vi "1D Quadrature Integrand for Gated Decay.vi"(10 "data":variant, 11 "X":dbl[](array[numeric])) -> (0 "Error Out":errorcluster, 3 "F(X)":dbl[](array[numeric]))   [LabVIEW 2019]
doc: "This template is the starting point for creating a function that is the integrand evaluation to be passed to the Quadrature.vi."
uses:
  Gate & Decay Parameters.ctl
  Gate Type.ctl
  IRF Model.ctl
  XY Plot Data.ctl
  a549e530-db8e-4861-84b1-6abd4ac2432e.vi/28aad339-045a-48ec-96ec-2fcecac66ea0.vi
  <vilib>/Utility/error.llb/Error Cluster From Error Code.vi
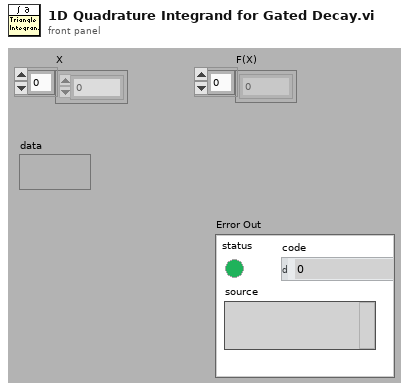
[diagram p1: front panel]
types:
  T1 = typedef "Gate & Decay Parameters.ctl" = cluster{"W":dbl, "T":dbl, "tau":dbl, "t_0":dbl, "Gate Type":T2, "t_i":dbl, "sR":dbl, "sF":dbl, "s":dbl, "Reversed Sawtooth":bool, "IRF Model":T3, "IRF Parameter 1":dbl, "User-defined Gate":T4, "Type of User-defined Function":enum32{"Gate", "IRF"}}
  T2 = typedef "Gate Type.ctl" = enum16{"Square", "Finite Edge Square", "Finite Edge, Tilted Top Square", "Triangle", "Sawtooth", "User-defined"}
  T3 = typedef "IRF Model.ctl" = enum16{"Dirac", "Exponential"}
  T4 = typedef "XY Plot Data.ctl" = cluster{"X Array":dbl[], "Y Array":dbl[]}
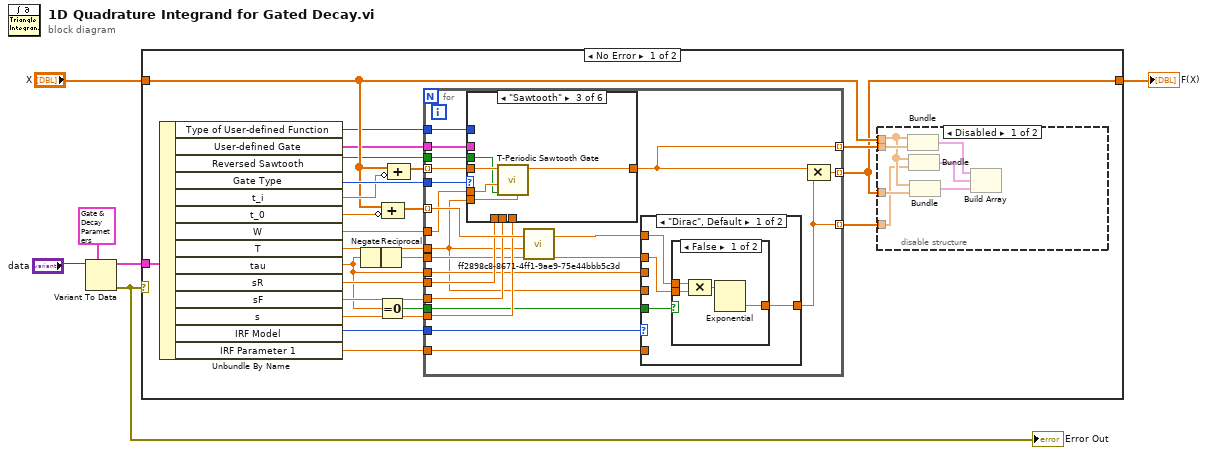
[diagram p0: block diagram]
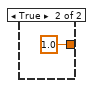
[diagram p3: hidden frame]
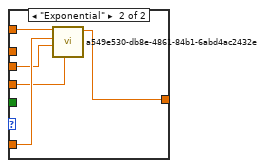
[diagram p4: hidden frame]
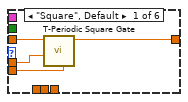
[diagram p5: hidden frame]
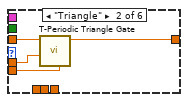
[diagram p6: hidden frame]
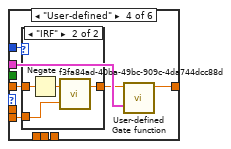
[diagram p7: hidden frame]
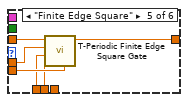
[diagram p9: hidden frame]
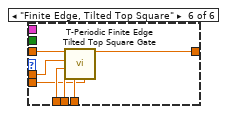
[diagram p10: hidden frame]
diagram:
  n1 = Variant To Data(type=T1 {"W"=0.0, "T"=0.0, "tau"=0.0, "t_0"=0.0, "Gate Type"=enum."Square", "t_i"=0.0, "sR"=0.0, "sF"=0.0, "s"=0.0, "Reversed Sawtooth"=FALSE, "IRF Model"=enum."Dirac", "IRF Parameter 1"=0.0, "User-defined Gate"={"X Array"=[], "Y Array"=[]}, "Type of User-defined Function"=enum."Gate"} ("Gate & Decay Parameters"), Variant="data") -> (data=w3:T1, error out=w2:errorcluster)  [unwired: 1 in]
  "Error Out" <- w2
  n2 = case shown="No Error" w2 {
    tunnel: "X" -> [w23 _]
    tunnel: w3 -> [w9 _]
    tunnel: [w7 _] -> w1
    frame No Error {
      n3 = Unbundle By Name(w9) -> ("Type of User-defined Function"=w8:enum32{"Gate", "IRF"}, "User-defined Gate"=w12:T4, "Reversed Sawtooth"=w15:bool, "Gate Type"=w29:T2, "t_i"=w28:dbl, "t_0"=w26:dbl, "W"=w21:dbl, "T"=w30:dbl, "tau"=w11:dbl, "sR"=w18:dbl, "sF"=w17:dbl, "s"=w16:dbl, "IRF Model"=w14:T3, "IRF Parameter 1"=w13:dbl)
      n4 = Negate(x=w11) -> (-x=w20:dbl)
      n5 = Reciprocal(x=w20) -> (1/x=w19:dbl)
      n6 = Equal To 0?(x=w11) -> (x = 0?=w10:bool)
      n7 = Compound Arithmetic op=ADD(w23, invert w26) -> (w25:dbl[])
      n8 = Compound Arithmetic op=ADD(w23, invert w28) -> (w27:dbl[])
      n9 = for {
        tunnel: w30 -> [w39]
        tunnel: w19 -> [w41]
        tunnel: w25 -> [w53] mode=indexing
        tunnel: w27 -> [w57] mode=indexing
        tunnel: w29 -> [w56]
        tunnel: [w55] -> w7 mode=indexing
        tunnel: [w54] -> w24 mode=indexing
        tunnel: [w51] -> w22 mode=indexing
        tunnel: w21 -> [w52]
        tunnel: w18 -> [w50]
        tunnel: w17 -> [w49]
        tunnel: w16 -> [w48]
        tunnel: w15 -> [w47]
        tunnel: w14 -> [w46]
        tunnel: w13 -> [w45]
        tunnel: w11 -> [w44]
        tunnel: w12 -> [w43]
        tunnel: w10 -> [w40]
        tunnel: w8 -> [w38]
        n10 = case shown="\"Sawtooth\"" w56 {
          tunnel: w52 -> [w74 w79 w83 _ w99 w106]
          tunnel: w57 -> [w75 w78 w84 w90 w101 w108]
          tunnel: [w73 w77 w82 w89 w100 w107] -> w54
          tunnel: w50 -> [_ _ _ _ w97 w105]
          tunnel: w49 -> [_ _ _ _ w96 w104]
          tunnel: w48 -> [_ _ _ _ _ w103]
          tunnel: w47 -> [_ _ w81 _ _ _]
          tunnel: w43 -> [_ _ _ w88 _ _]
          tunnel: w39 -> [w72 w76 w80 w87 w98 w102]
          tunnel: w38 -> [_ _ _ w85 _ _]
          frame "Square", Default {
            n11 = call "T-Periodic Square Gate.vi"("Period T"=w72, "W"=w74, "t"=w75) -> ("Square(t)"=w73:dbl)  [unwired: 8 in]
          }
          frame "Triangle" {
            n12 = call "T-Periodic Triangle Gate.vi"("Period T"=w76, "W"=w79, "t"=w78) -> ("Triangle(t)"=w77:dbl)  [unwired: 8 in]
          }
          frame "Sawtooth" {
            n13 = call "T-Periodic Sawtooth Gate.vi"("Period T"=w80, "Reversed?"=w81, "W"=w83, "t"=w84) -> ("Sawtooth(t)"=w82:dbl)  [unwired: 7 in]
          }
          frame "User-defined" {
            n14 = case shown="\"IRF\"" w85 {
              tunnel: w90 -> [w91 w95]
              tunnel: w87 -> [_ w93]
              tunnel: [w91 w92] -> w86
              frame "Gate", Default {
              }
              frame "IRF" {
                n15 = Negate(x=w95) -> (-x=w94:dbl)
                n16 = call "f3fa84ad-40ba-49bc-909c-4da744dcc88d.vi"("y"=w93, "x"=w94) -> ("x - E(x/y)y"=w92:dbl)  [unwired: 1 out]
              }
            }
            n17 = call "User-defined Gate function.vi"("User-defined Gate"=w88, "t"=w86) -> ("User-defined Gate(t)"=w89:dbl)  [unwired: 8 in, 1 out]
          }
          frame "Finite Edge Square" {
            n18 = call "T-Periodic Finite Edge Square Gate.vi"("Period T"=w98, "s_F"=w96, "s_R"=w97, "W"=w99, "t"=w101) -> ("Finite Edge Square(t)"=w100:dbl)  [unwired: 6 in]
          }
          frame "Finite Edge, Tilted Top Square" {
            n19 = call "T-Periodic Finite Edge Tilted Top Square Gate.vi"("Period T"=w102, "slope"=w103, "s_F"=w104, "s_R"=w105, "W"=w106, "t"=w108) -> ("Finite Edge Square(t)"=w107:dbl)  [unwired: 5 in]
          }
        }
        n20 = call "ff2898c8-8671-4ff1-9ae9-75e44bbb5c3d.vi"("y"=w39, "x"=w53) -> ("x - E(x/y)y"=w42:dbl)  [unwired: 1 out]
        n21 = case shown="\"Dirac\", Default" w46 {
          tunnel: [w60 w70] -> w51
          tunnel: w42 -> [w59 w71]
          tunnel: w45 -> [_ w69]
          tunnel: w44 -> [_ w68]
          tunnel: w39 -> [_ w67]
          tunnel: w41 -> [w61 _]
          tunnel: w40 -> [w58 _]
          frame "Dirac", Default {
            n22 = case shown="False" w58 {
              tunnel: w61 -> [w65 _]
              tunnel: [w64 1.0] -> w60
              tunnel: w59 -> [w63 _]
              frame False {
                n23 = Compound Arithmetic op=MULTIPLY(w63, w65) -> (w62:dbl)
                n24 = Exponential(1:w62) -> (0:w64:dbl)
              }
              frame True {
              }
            }
          }
          frame "Exponential" {
            n25 = call "a549e530-db8e-4861-84b1-6abd4ac2432e.vi"("Period: T"=w67, "lifetime: tau"=w68, "IRF time constant"=w69, "t"=w71) -> ("y(t)"=w70:dbl)  [unwired: 6 in, 1 out]
          }
        }
        n26 = Compound Arithmetic op=MULTIPLY(w54, w51) -> (w55:dbl)
      }
      n27 = disable-structure shown="Disabled" {
        disable-tunnel: w7 -> [w37 _]
        disable-tunnel: w24 -> [w35 _]
        disable-tunnel: w23 -> [w34 _]
        disable-tunnel: w22 -> [w33 _]
        frame Disabled {
          n28 = Bundle("X"=w34, w35) -> (w32:cluster{"X":dbl[], dbl[]})  [unwired: 1 in]
          n29 = Bundle("X"=w34, w33) -> (w31:cluster{"X":dbl[], dbl[]})  [unwired: 1 in]
          n30 = Bundle("X"=w34, w37) -> (w36:cluster{"X":dbl[], dbl[]})  [unwired: 1 in]
          n31 = Build Array(w32, w31, w36) -> ()  [unwired: 1 out]
        }
        frame Enabled {
        }
      }
    }
    frame Error {
    }
  }
  "F(X)" <- w1
